vi "PCert-ConfigPageNF-ChangeActiveConnectionDB.vi"(8 "error in (no error)":errorcluster, 10 "Plugin Caller":refnum<class "FTW-ActorConnector.lvclass">, 11 "ERP-ConfigPageNF in":refnum<class "PCert-ConfigPageNF.lvclass">) -> (0 "error out":errorcluster, 3 "ERP-ConfigPageNF out":refnum<class "PCert-ConfigPageNF.lvclass">)   [LabVIEW 2013, in "PCert-ConfigPageNF.lvclass"]
uses:
  PCert-ConfigPageNF.lvclass
  ftw-dataflow/Actor/src/Connector/FTW-ActorConnector.lvclass
  PCert-ConfigPageNF.lvclass/PCert-ConfigPageNF.ctl
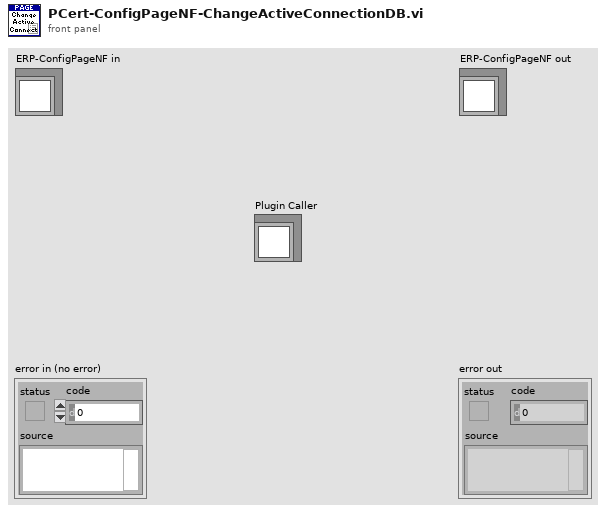
[diagram p1: front panel]
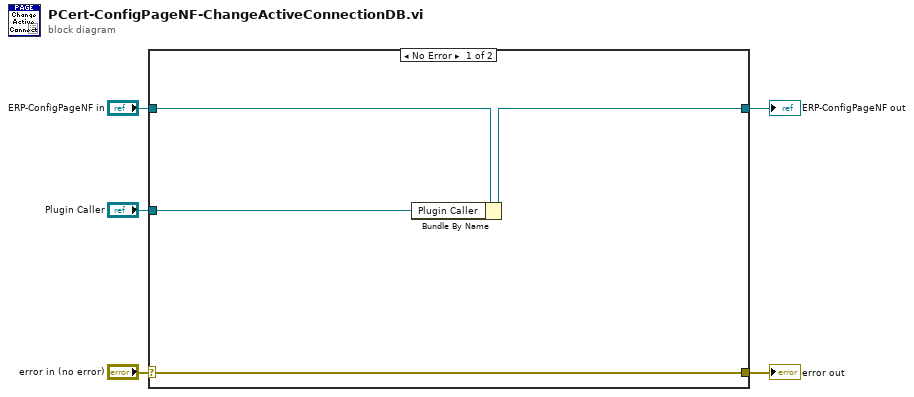
[diagram p0: block diagram]
diagram:
  n1 = case shown="No Error" "error in (no error)" {
    selector: "error in (no error)" -> [w9 w11]
    tunnel: [w9 w11] -> w4
    tunnel: [w7 w10] -> w2
    tunnel: "ERP-ConfigPageNF in" -> [w8 w10]
    tunnel: "Plugin Caller" -> [w6 _]
    frame No Error {
      n2 = Bundle By Name(cluster=w8, "Plugin Caller"=w6) -> (w7:refnum<class "PCert-ConfigPageNF.lvclass">)
    }
    frame Error {
    }
  }
  "error out" <- w4
  "ERP-ConfigPageNF out" <- w2
